vi "数据查询_仪器数据.vi"() -> ()   [LabVIEW 2016]
uses:
  <vilib>/Utility/miscctls.llb/LVRowAndColumnUnsignedTypeDef.ctl
  <vilib>/Utility/miscctls.llb/LVPointTypeDef.ctl
  <userlib>/_OpenG.lib/array/array.llb/Sort 2D Array (String)__ogtk.vi
panel:
  out "布尔":bool
  in  "页":i32 format="第%.0f页"
  in  "每页条数":i32=20
  in  "向后按钮":bool
  in  "向前按钮":bool
  in  "下拉列表":string(xcontrol)
  in  "导出":bool
  out "分钟小时":string(combo)="实时数据"
  out "工作类型":string(combo)="全部数据"
  in  "查询":bool
  in  "结束日期":string="2050/01/01"
  in  "起始日期":string="2010/01/01"
  out "数据表":string[][](table)
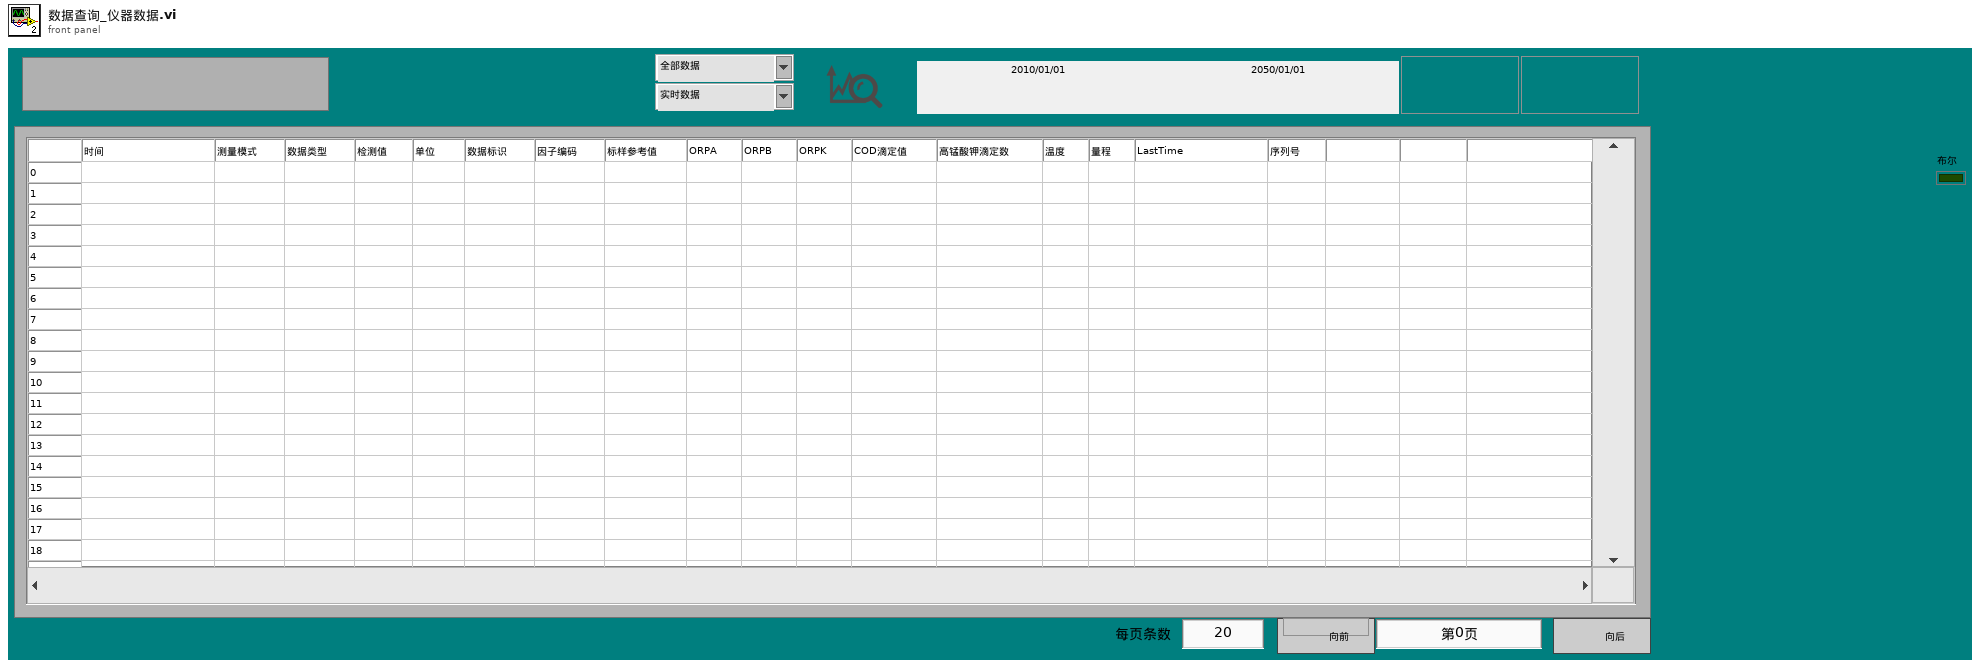
[diagram p1: front panel]
types:
  T1 = enum8{"Enabled", "Disabled", "Disabled and Grayed Out"}
  T2 = typedef "LVRowAndColumnUnsignedTypeDef.ctl" = cluster{"Row":u32, "Column":u32}
  T3 = typedef "LVPointTypeDef.ctl" = cluster{"Horizontal":i16, "Vertical":i16}
  T4 = typedef "LVDateTimeRec.ctl" = cluster{"秒数的小数部分":dbl, "秒":i32, "分":i32, "时":i32, "日":i32, "月":i32, "年":i32, "天数（周）":i32, "天数（年）":i32, "DST":i32}
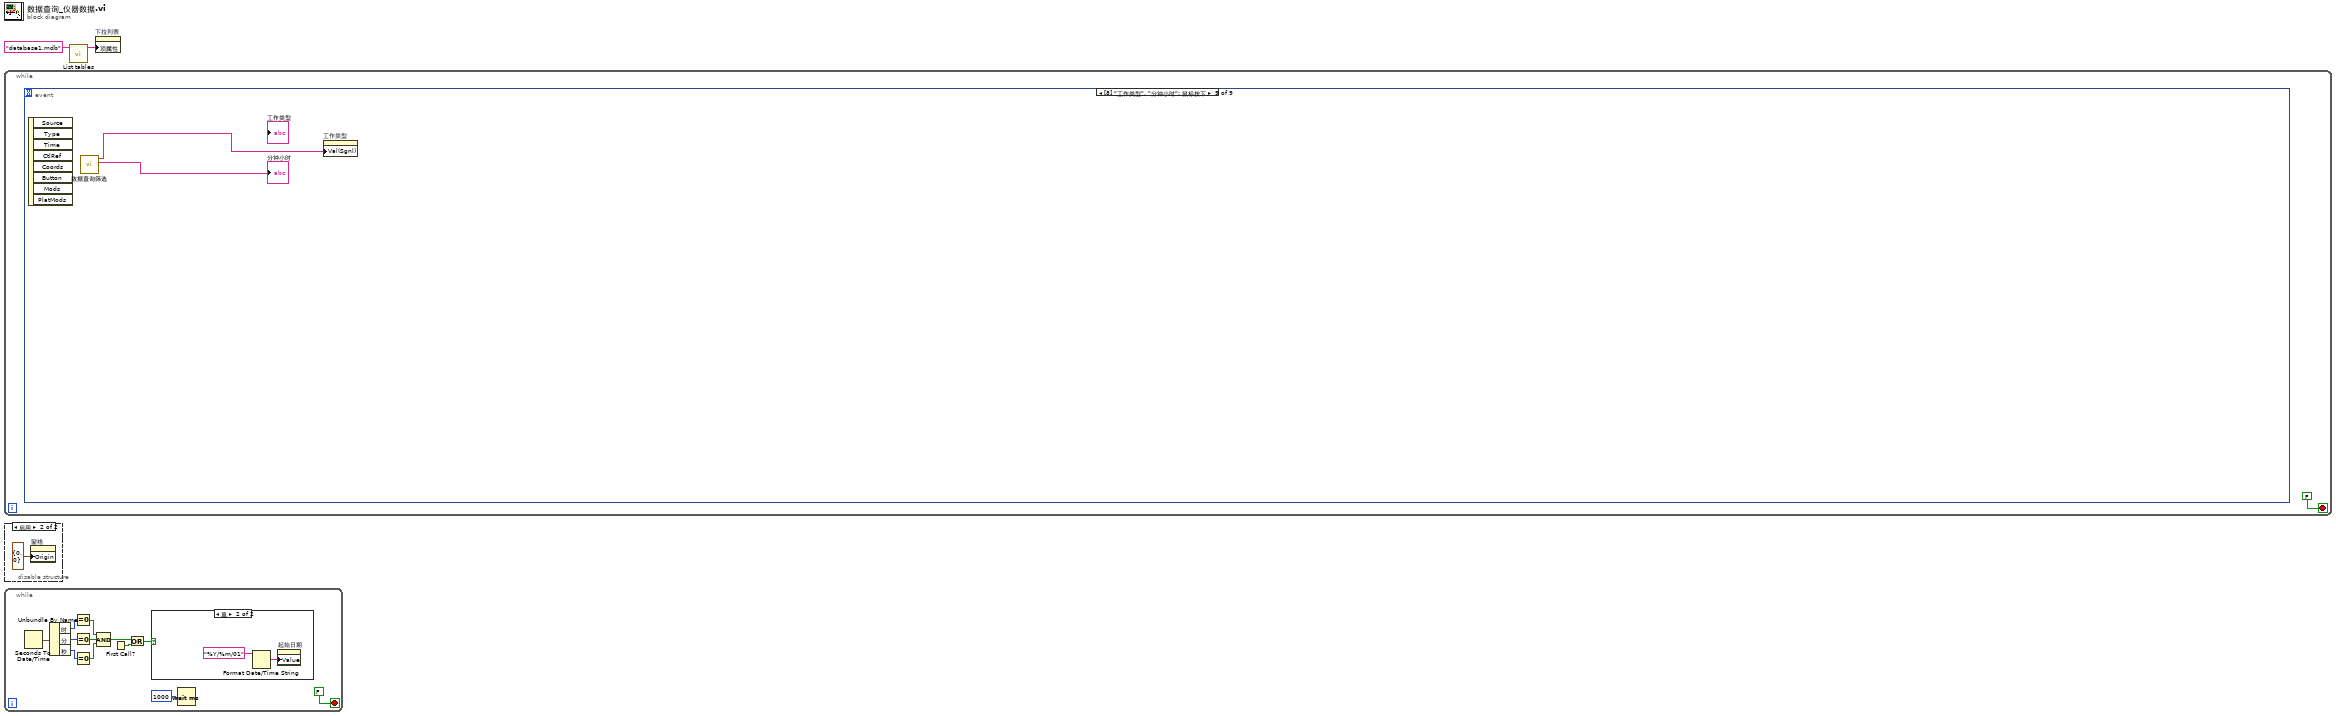
[diagram p0: block diagram]
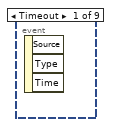
[diagram p3: hidden frame]
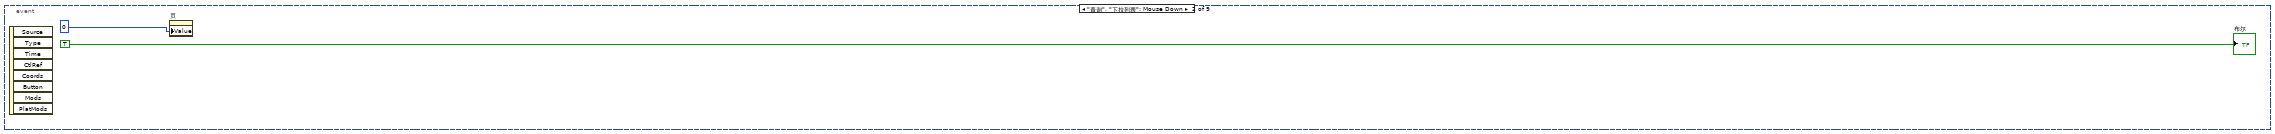
[diagram p4: hidden frame]
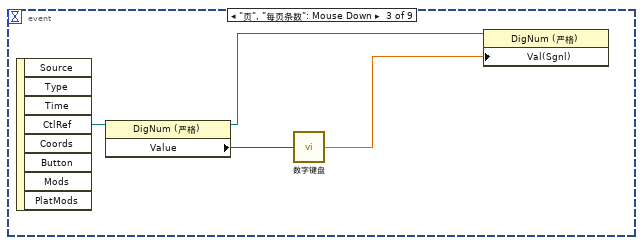
[diagram p5: hidden frame]
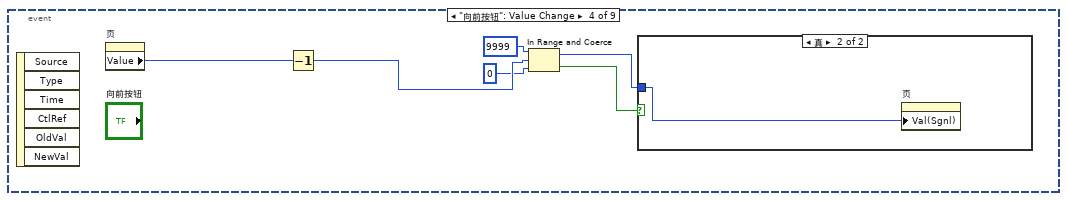
[diagram p6: hidden frame]
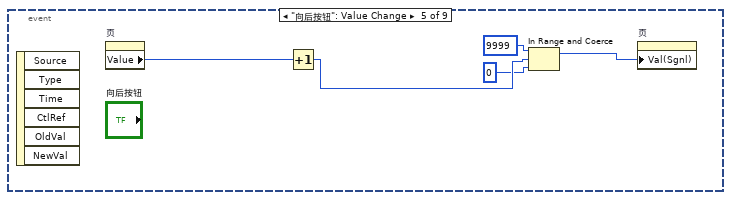
[diagram p8: hidden frame]
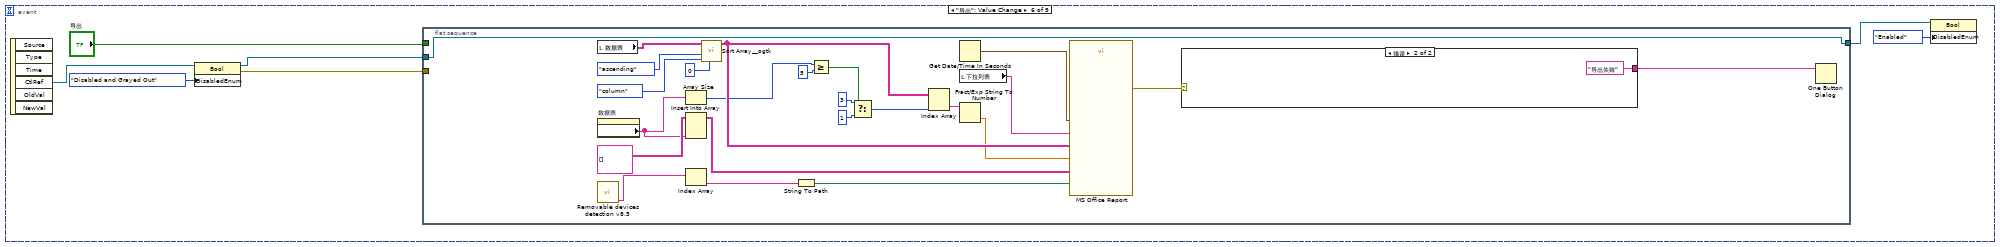
[diagram p9: hidden frame]
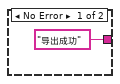
[diagram p10: hidden frame]
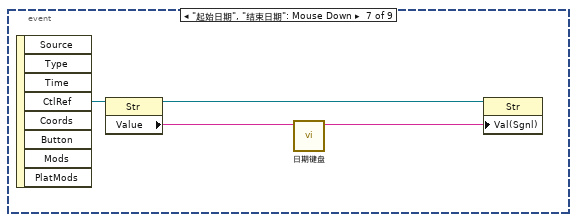
[diagram p11: hidden frame]
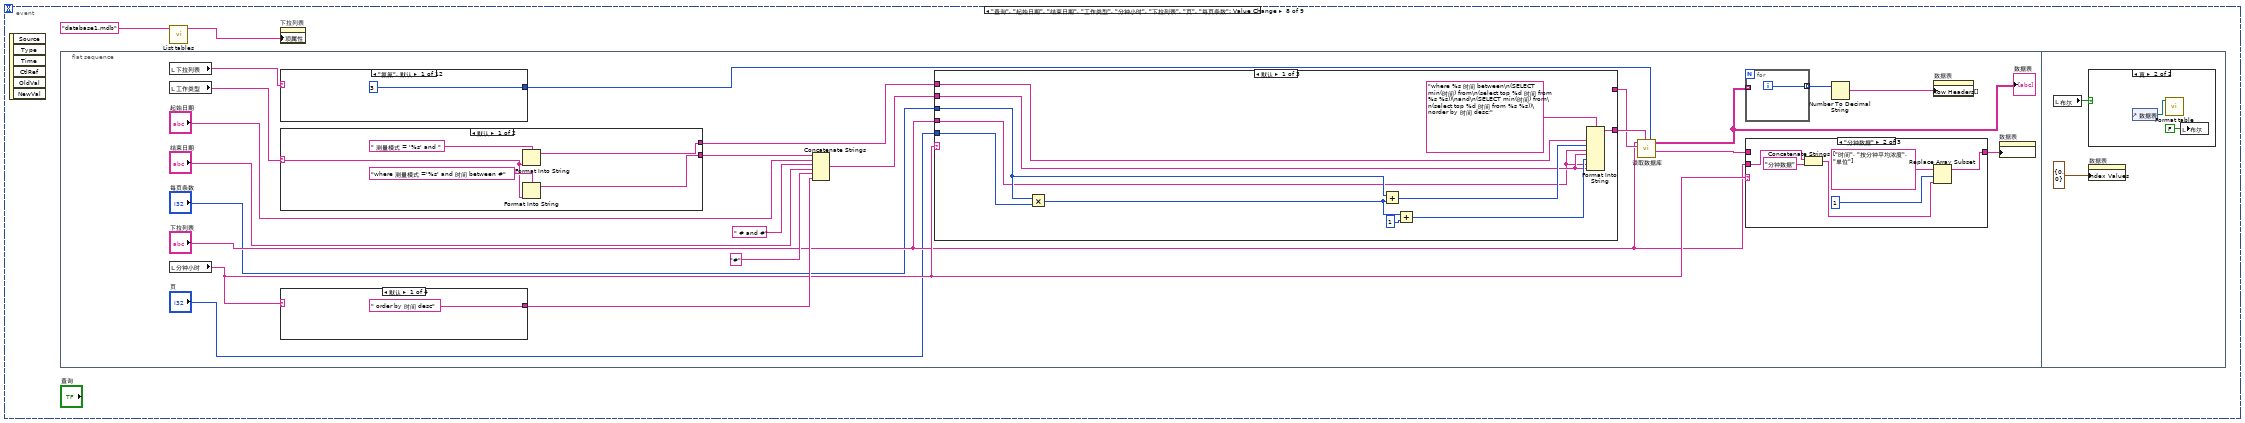
[diagram p12: hidden frame]
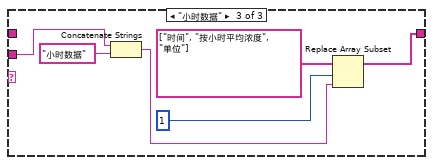
[diagram p14: hidden frame]
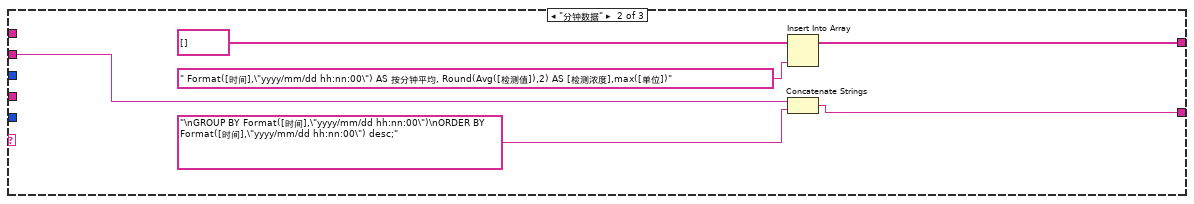
[diagram p18: hidden frame]
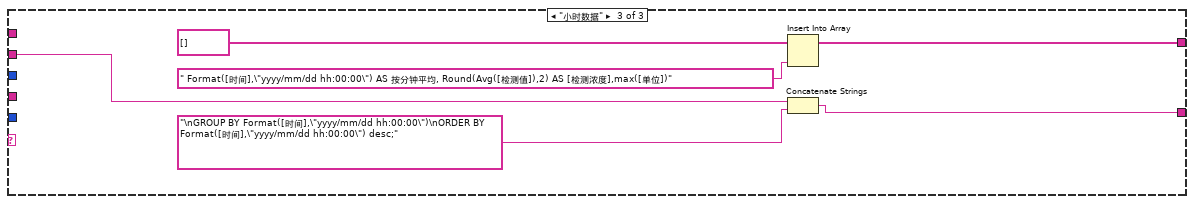
[diagram p19: hidden frame]
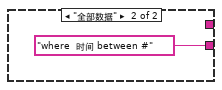
[diagram p20: hidden frame]
diagram:
  n1 = while {
    stop <- FALSE stop-if-true
    n2 = event shown="[8] \"工作类型\", \"分钟小时\": 鼠标按下" {
      selector: _ -> [_ _ _ _ _ _ _ _ _]
      dyn-events: _ -> [_ _ _ _ _ _ _ _ _]
      timeout: _ -> [_ _ _ _ _ _ _ _ _]
      event Timeout {
        n3 = event-data() -> ()  [unwired: 1 in, 3 out]
      }
      event "查询", "下拉列表": Mouse Down {
        n4 = event-data() -> ()  [unwired: 1 in, 8 out]
        n5 = property on="页" class="DigNum (严格)"("Value"=0 ("页")) -> ()  [unwired: 2 in, 2 out]
        "布尔" <- TRUE ("布尔")
      }
      event "页", "每页条数": Mouse Down {
        n6 = event-data() -> ("CtlRef"=w6:refnum<vi>)  [unwired: 1 in, 7 out]
        n7 = property class="DigNum (严格)"(reference=w6) -> (reference out=w7:refnum<vi>, "Value"=w9:i32)  [unwired: 1 in, 1 out]
        n8 = call "数字键盘.vi"("OldNumber"=w9) -> ("NewNumber"=w8:sgl)
        n9 = property class="DigNum (严格)"(reference=w7, "Val(Sgnl)"=w8) -> ()  [unwired: 1 in, 2 out]
      }
      event "向前按钮": Value Change {
        n10 = event-data() -> ()  [unwired: 1 in, 6 out]
        n11 = property on="页" class="DigNum (严格)"() -> ("Value"=w15:i32)  [unwired: 2 in, 2 out]
        n12 = Decrement(x=w15) -> (x-1=w14:i32)
        n13 = In Range and Coerce(upper limit=9999 ("上限"), x=w14, lower limit=0 ("下限")) -> (coerced(x)=w11:i32, In Range?=w10:bool)
        n14 = case shown="真" w10 {
          tunnel: w11 -> [_ w16]
          frame False {
          }
          frame True {
            n15 = property on="页" class="DigNum (严格)"("Val(Sgnl)"=w16) -> ()  [unwired: 2 in, 2 out]
          }
        }
      }
      event "向后按钮": Value Change {
        n16 = event-data() -> ()  [unwired: 1 in, 6 out]
        n17 = property on="页" class="DigNum (严格)"() -> ("Value"=w21:i32)  [unwired: 2 in, 2 out]
        n18 = Increment(x=w21) -> (x+1=w20:i32)
        n19 = In Range and Coerce(upper limit=u32 9999 ("上限"), x=w20, lower limit=u32 0 ("下限")) -> (coerced(x)=w17:u32)  [unwired: 1 out]
        n20 = property on="页" class="DigNum (严格)"("Val(Sgnl)"=w17) -> ()  [unwired: 2 in, 2 out]
      }
      event "导出": Value Change {
        n21 = event-data() -> ("CtlRef"=w22:refnum<vi>)  [unwired: 1 in, 5 out]
        n22 = property class="Bool"(reference=w22, "DisabledEnum"=T1."Disabled and Grayed Out" ("禁用")) -> (reference out=w26:refnum<vi>, error out=w27:errorcluster)  [unwired: 1 in]
        n23 = flat-sequence {
          tunnel: w27 -> [_]
          tunnel: [w43] -> w25
          tunnel: w26 -> [w43]
          tunnel: "导出" -> [_]
          frame #0 {
            n24 = local read "数据表"() -> (w51:string[][])
            n25 = property on="数据表" class="Tbl (严格)"() -> ("Column Headers[]"=w30:string[])  [unwired: 2 in, 2 out]
            n26 = call "Removable devices detection v8.5.vi"() -> ("Removable"=w40:string[])  [unwired: 4 out]
            n27 = Array Size(array=w30) -> (size(s)=w37:i32)
            n28 = Insert Into Array(array=string[][] [], new element=w30) -> (w29:string[][])  [unwired: 2 in]
            n29 = Index Array(array=w40) -> (element=w39:string)  [unwired: 1 in]
            n30 = call-poly <userlib>:"Sort Array__ogtk.vi"("Column/Row to Sort By"=u32 0, "Sort By in"=enum16{"row", "column"}."column", "Order"=enum16{"ascending", "descending"}."ascending", "Array in"=w51) -> ("Sorted Array out"=w50:string[][])  [unwired: 4 in, 3 out]
            n31 = String To Path(string=w39) -> (path=w38:path)
            n32 = Greater Or Equal?(x=w37, y=5) -> (x >= y?=w35:bool)
            n33 = Select(t=3 ("禁用的索引 (列)"), s=w35, f=1) -> (s? t:f=w33:i32)
            n34 = Index Array(array=w50, index (col)=w33) -> (element=w46:string[])  [unwired: 1 in]
            n35 = Get Date/Time In Seconds() -> (seconds since 1Jan1904=w52:timestamp)
            n36 = local read "下拉列表"() -> (w44:string)
            n37 = Fract/Exp String To Number(string=w46) -> (number=w45:dbl[])  [unwired: 3 in, 1 out]
            n38 = call "MS Office Report"("Path to Save Report"=w38, "导出日期"=w52, "监测参数"=w44, "数据输入"=w50, "图表输入"=w45, "字段定义"=w29) -> ("error out"=w42:errorcluster)  [unwired: 20 in, 1 out]
            n39 = case shown="错误" w42 {
              tunnel: ["导出成功" ("消息") "导出失败" ("消息")] -> w41
              frame No Error {
              }
              frame Error {
              }
            }
            n40 = One Button Dialog(message=w41) -> ()  [unwired: 1 in, 1 out]
          }
        }
        n41 = property class="Bool"(reference=w25, "DisabledEnum"=T1."Enabled" ("禁用")) -> ()  [unwired: 1 in, 2 out]
      }
      event "起始日期", "结束日期": Mouse Down {
        n42 = event-data() -> ("CtlRef"=w58:refnum<vi>)  [unwired: 1 in, 7 out]
        n43 = property class="Str"(reference=w58) -> (reference out=w56:refnum<vi>, "Value"=w57:string)  [unwired: 1 in, 1 out]
        n44 = call "日期键盘.vi"("原值"=w57) -> ("x+y"=w55:string)  [unwired: 10 in]
        n45 = property class="Str"(reference=w56, "Val(Sgnl)"=w55) -> ()  [unwired: 1 in, 2 out]
      }
      event "查询", "起始日期", "结束日期", "工作类型", "分钟小时", "下拉列表", "页", "每页条数": Value Change {
        n46 = event-data() -> ()  [unwired: 1 in, 6 out]
        n47 = flat-sequence {
          frame #0 {
            n48 = local read "下拉列表"() -> (w75:string)
            n49 = local read "工作类型"() -> (w73:string)
            n50 = local read "分钟小时"() -> (w67:string)
            n51 = case shown="\"氨氮\", 默认" w75 {
              tunnel: [i16 3 ("精度(6)") i16 1 ("精度(6)") i16 2 ("精度(6)") i16 2 ("精度(6)") i16 2 ("精度(6)") i16 2 ("精度(6)") i16 2 ("精度(6)") i16 2 ("精度(6)") i16 3 ("精度(6)") i16 2 ("精度(6)") i16 2 ("精度(6)") i16 2 ("精度(6)")] -> w74
              frame "氨氮", Default {
              }
              frame "水温" {
              }
              frame "pH" {
              }
              frame "溶解氧" {
              }
              frame "电导率" {
              }
              frame "浊度" {
              }
              frame "藻密度" {
              }
              frame "叶绿素a" {
              }
              frame "总磷" {
              }
              frame "总氮" {
              }
              frame "CodCr" {
              }
              frame "CodMn" {
              }
            }
            n52 = case shown="默认" w73 {
              selector: w73 -> [w121 _]
              tunnel: [w123 "where  时间 between #" ("condition")] -> w72
              tunnel: [w120 _] -> w61
              frame Default {
                n53 = Format Into String(format string=" 测量模式 = '%s' and " ("condition"), w121) -> (resulting string=w120:string)  [unwired: 2 in, 1 out]
                n54 = Format Into String(format string="where 测量模式 ='%s' and 时间 between #" ("condition"), w121) -> (resulting string=w123:string)  [unwired: 2 in, 1 out]
              }
              frame "全部数据" {
              }
            }
            n55 = case shown="默认" w67 {
              tunnel: [" order by 时间 desc" ("字符串") _ _ _] -> w71
              frame Default {
              }
              frame "分钟数据" {
              }
              frame "小时数据" {
              }
              frame "真" {
              }
            }
            n56 = Concatenate Strings(w72, "起始日期", " # and #" ("condition"), "结束日期", "#" ("condition"), w71) -> (w70:string)
            n57 = case shown="默认" w67 {
              tunnel: [_ w112 w114] -> w68
              tunnel: w70 -> [w99 w110 w116]
              tunnel: [w102 w109 w115] -> w69
              tunnel: "下拉列表" -> [w98 _ _]
              tunnel: "每页条数" -> [w101 _ _]
              tunnel: "页" -> [w100 _ _]
              tunnel: w61 -> [w97 _ _]
              frame Default {
                n58 = Multiply(x=w101, y=w100) -> (x*y=w106:i32)
                n59 = Add(x=w101, y=w106) -> (x+y=w104:i32)
                n60 = Add(x=w106, y=u32 1) -> (x+y=w103:u32)
                n61 = Format Into String(format string="where %s 时间 between\n(SELECT min(时间) from\n(select top %d 时间 from %s %s))\nand\n(SELECT min(时间) from\n(select top %d 时间 from %s %s))\norder by 时间 desc;" ("格式字符串"), w97, w104, w98, w99, w103, w98, w99) -> (resulting string=w102:string)  [unwired: 2 in, 1 out]
              }
              frame "分钟数据" {
                n62 = Insert Into Array(array=string[] [] ("显示项"), new element=" Format([时间],\"yyyy/mm/dd hh:nn:00\") AS 按分钟平均, Round(Avg([检测值]),2) AS [检测浓度],max([单位])" ("新元素/子数组")) -> (w112:string[])  [unwired: 1 in]
                n63 = Concatenate Strings(w110, "\nGROUP BY Format([时间],\"yyyy/mm/dd hh:nn:00\")\nORDER BY Format([时间],\"yyyy/mm/dd hh:nn:00\") desc;" ("字符串")) -> (w109:string)
              }
              frame "小时数据" {
                n64 = Insert Into Array(array=string[] [] ("显示项"), new element=" Format([时间],\"yyyy/mm/dd hh:00:00\") AS 按分钟平均, Round(Avg([检测值]),2) AS [检测浓度],max([单位])" ("新元素/子数组")) -> (w114:string[])  [unwired: 1 in]
                n65 = Concatenate Strings(w116, "\nGROUP BY Format([时间],\"yyyy/mm/dd hh:00:00\")\nORDER BY Format([时间],\"yyyy/mm/dd hh:00:00\") desc;" ("字符串")) -> (w115:string)
              }
            }
            n66 = call "读取数据库.vi"("精度(6)"=w74, "condition"=w69, "显示项"=w68, "组合框"="下拉列表") -> ("columns"=w66:string[], "表格"=w78:string[][])  [unwired: 4 in, 2 out]
            "数据表" <- w78
            n67 = for {
              tunnel: w78 -> [_] mode=indexing
              tunnel: [w138] -> w77 mode=indexing
              i -> [w138]
            }
            n68 = case shown="\"分钟数据\"" w67 {
              tunnel: w66 -> [w83 _ _]
              tunnel: [w83 w87 w91] -> w65
              tunnel: "下拉列表" -> [_ w86 w92]
              frame Default {
              }
              frame "分钟数据" {
                n69 = Concatenate Strings(w86, "分钟数据" ("字符串")) -> (w84:string)
                n70 = Replace Array Subset(array=string[] ["时间", "按分钟平均浓度", "单位"] ("columns"), new element=w84, index=1 ("索引")) -> (w87:string[])
              }
              frame "小时数据" {
                n71 = Concatenate Strings(w92, "小时数据" ("字符串")) -> (w93:string)
                n72 = Replace Array Subset(array=string[] ["时间", "按小时平均浓度", "单位"] ("columns"), new element=w93, index=1 ("索引")) -> (w91:string[])
              }
            }
            n73 = Number To Decimal String(number=w77) -> (decimal integer string=w76:string[])  [unwired: 1 in]
            n74 = property on="数据表" class="Tbl (严格)"("Row Headers[]"=w76) -> ()  [unwired: 2 in, 2 out]
            n75 = property on="数据表" class="Tbl (严格)"("Column Headers[]"=w65) -> ()  [unwired: 2 in, 2 out]
          }
          frame #1 {
            n76 = local read "布尔"() -> (w139:bool)
            n77 = case shown="真" w139 {
              frame False {
              }
              frame True {
                n78 = control-ref of="数据表"() -> (w142:refnum<vi>)
                n79 = call "Format table.vi"("Table输入"=w142) -> ()  [unwired: 11 in]
                n80 = local write "布尔"(FALSE ("布尔")) -> ()
              }
            }
            n81 = property on="数据表" class="Tbl (严格)"("Index Values"=T2 {"Row"=0, "Column"=0} ("索引值")) -> ()  [unwired: 2 in, 2 out]
          }
        }
        n82 = call "List tables.vi"("database"="database1.mdb") -> ("tables"=w59:string[])  [unwired: 9 in, 1 out]
        n83 = property on="下拉列表" class="下拉列表 (严格)"("项属性"=w59) -> ()  [unwired: 2 in, 2 out]
      }
      event "工作类型", "分钟小时": Mouse Down {
        n84 = event-data() -> ()  [unwired: 1 in, 8 out]
        n85 = call "数据查询筛选.vi"() -> ("分钟小时"=→"分钟小时":string, "工作类型"=w143:string)  [unwired: 10 in]
        n86 = property on="工作类型" class="CmbBox"("Val(Sgnl)"=w143) -> ()  [unwired: 2 in, 2 out]
      }
    }
  }
  n87 = disable-structure shown="启用" {
    frame Disabled {
    }
    frame Enabled {
      n88 = property on="窗格" class="Pane"("Origin"=T3 {"Horizontal"=0, "Vertical"=0} ("原点")) -> ()  [unwired: 2 in, 2 out]
    }
  }
  n89 = while {
    stop <- FALSE stop-if-true
    n90 = Seconds To Date/Time() -> (date time rec=w157:T4)  [unwired: 2 in]
    n91 = Unbundle By Name(w157) -> ("时"=w156:i32, "分"=w155:i32, "秒"=w154:i32)
    n92 = Equal To 0?(x=w156) -> (x = 0?=w153:bool)
    n93 = Equal To 0?(x=w155) -> (x = 0?=w152:bool)
    n94 = Equal To 0?(x=w154) -> (x = 0?=w151:bool)
    n95 = Compound Arithmetic op=AND ("复合运算")(w153, w152, w151) -> (w148:bool)
    n96 = First Call?() -> (First Call?: T/F=w146:bool)
    n97 = Or(x=w148, y=w146) -> (x .or. y?=w147:bool)
    n98 = case shown="真" w147 {
      frame False {
      }
      frame True {
        n99 = Format Date/Time String(time format string (%c)="%Y/%m/01" ("时间格式字符串(%c)")) -> (date/time string=w158:string)  [unwired: 2 in]
        n100 = property on="起始日期" class="Str"("Value"=w158) -> ()  [unwired: 2 in, 2 out]
      }
    }
    n101 = Wait (ms)(milliseconds to wait=u32 1000 ("等待时间（毫秒）")) -> ()  [unwired: 1 out]
  }
  n102 = call "List tables.vi"("database"="database1.mdb") -> ("tables"=w1:string[])  [unwired: 9 in, 1 out]
  n103 = property on="下拉列表" class="下拉列表 (严格)"("项属性"=w1) -> ()  [unwired: 2 in, 2 out]
